vi "Compute Distance.vi"(6 "Camera Info":T1, 8 "Height from camera of target":dbl, 10 "Bounding Box":T2) -> (2 "Bounding Box (Rad)":T2, 3 "Distance to target [in 2-space]":dbl)   [LabVIEW 2012]
doc: "Using the camera lens information and the real world width of the target, determine the distance to the target."
uses:
  CameraResolutionInfo.ctl
panel:
  in  "Camera angle offset (deg)":dbl
  # "Note:  '2-space' means that\nthis is not the absolute distance\nfrom the camera, but actually the distance\nfrom the camera to the target parallel to the\nfloor."
  # "ORIGINAL\n48\n43.5"
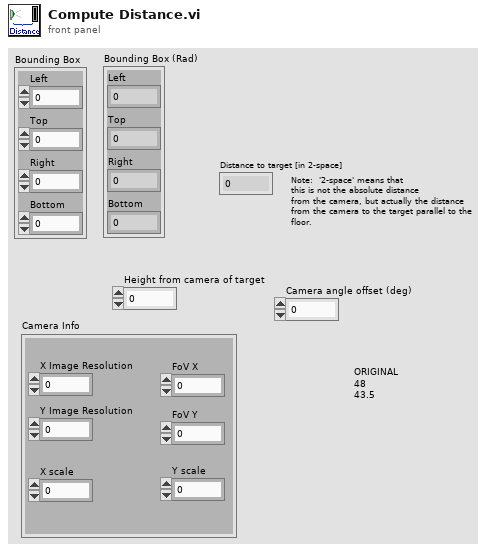
[diagram p1: front panel]
types:
  T1 = typedef "CameraResolutionInfo.ctl" = cluster{"X Image Resolution":i32, "Y Image Resolution":i32, "FoV X":dbl, "FoV Y":dbl, "X scale":dbl, "Y scale":dbl}
  T2 = cluster{"Left":dbl, "Top":dbl, "Right":dbl, "Bottom":dbl}
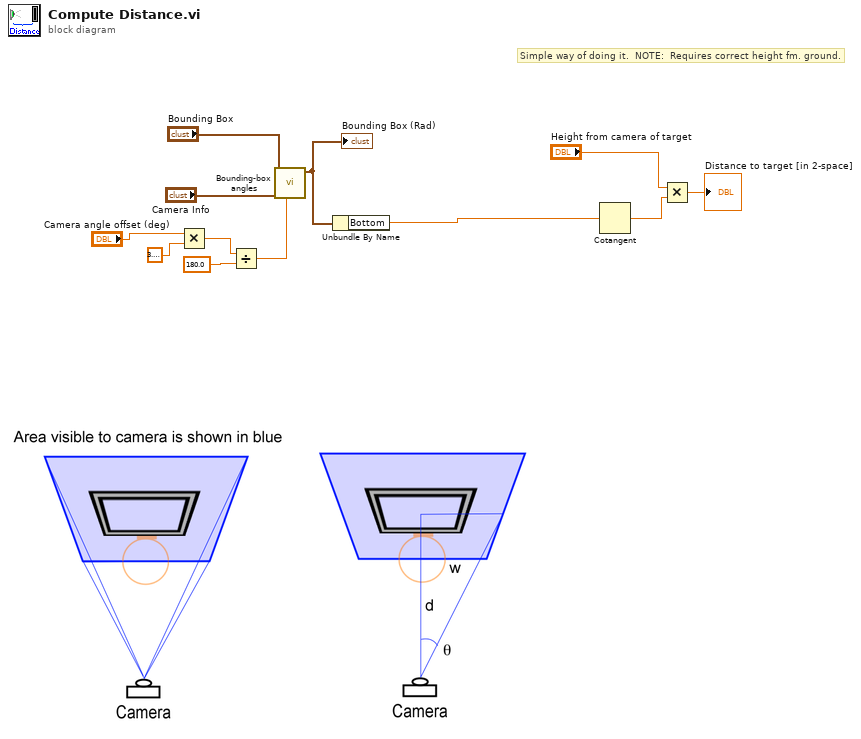
[diagram p0: block diagram]
diagram:
  # "Simple way of doing it.  NOTE:  Requires correct height fm. ground."
  n1 = Multiply(x="Camera angle offset (deg)", y=3.141592653589793) -> (x*y=w5:dbl)
  n2 = Divide(x=w5, y=180.0) -> (x/y=w4:dbl)
  n3 = call "Bounding-box angles.vi"("Camera angle offset (rad)"=w4, "Camera Info"="Camera Info", "Bounding Box"="Bounding Box") -> ("Bounding box (radians)"=w10:T2)  [unwired: 8 in]
  "Bounding Box (Rad)" <- w10
  n4 = Unbundle By Name(w10) -> ("Bottom"=w9:dbl)
  n5 = Cotangent(1:w9) -> (0:w3:dbl)
  n6 = Multiply(x="Height from camera of target", y=w3) -> (x*y=→"Distance to target [in 2-space]":dbl)
